vi "Degrees Minutes Seconds to Decimal.vi"(9 "Seconds":dbl format="%#.5g", 10 "Minutes":dbl, 11 "Degrees":dbl) -> (3 "Lat Long Input (decimal)":dbl format="%#.7g")   [LabVIEW 2014]
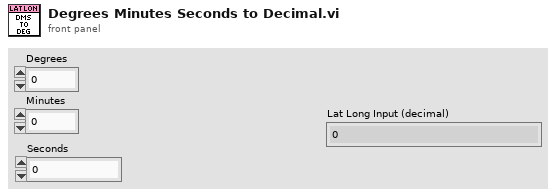
[diagram p1: front panel]
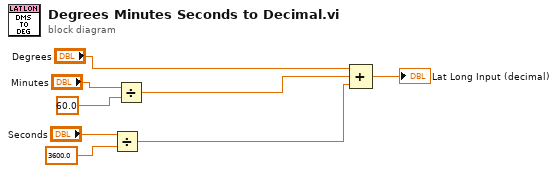
[diagram p0: block diagram]
diagram:
  n1 = Divide(x="Seconds", y=3600.0) -> (x/y=w2:dbl)
  n2 = Divide(x="Minutes", y=60.0) -> (x/y=w3:dbl)
  n3 = Compound Arithmetic op=ADD("Degrees", w3, w2) -> (→"Lat Long Input (decimal)":dbl)
